vi "Google - Raw Stock Data - Parse.vi"(0 "Raw Stock Data":string, 3 "error in":errorcluster) -> (7 "Stock Data":T1, 10 "error out":errorcluster)   [LabVIEW 2011]
doc: "Parse the Raw Stock Data to a cluster structure.\n\nInputs:\n Raw Stock Data: Body of the HTTP request.\n Error in: Describes error conditions that occur before this node runs. This input provides standard error in functionality.\n\nOutputs:\n Stock Data: Parsed Stock Data\n Symbol\n Name\n Price\n Change\n Change %\n Volume: N/A\n Error out: Contains error information. This output provides standard error out functionality."
uses:
  Stock Data Control.ctl
panel:
  out "Raw Data":string
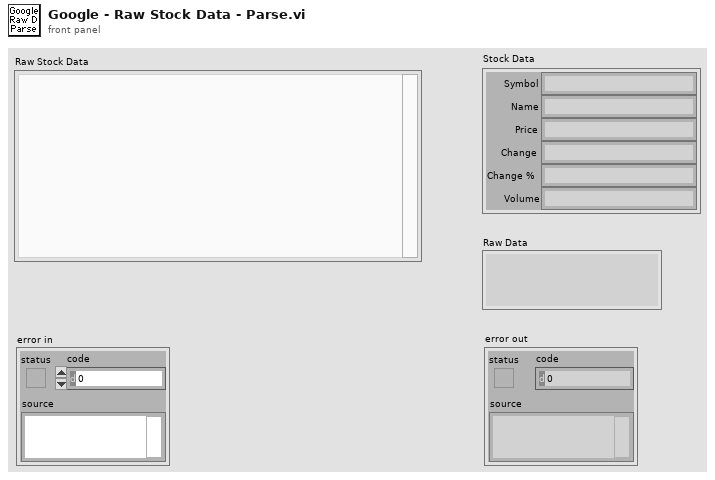
[diagram p1: front panel]
types:
  T1 = typedef "Stock Data Control.ctl" = cluster{"Symbol":string, "Name":string, "Price":string, "Change":string, "Change %":string, "Volume":string}
  T2 = cluster{"Symbol":string, "Name":string, "Price":string, "Change":string, "Change %":string, "Volume":string}
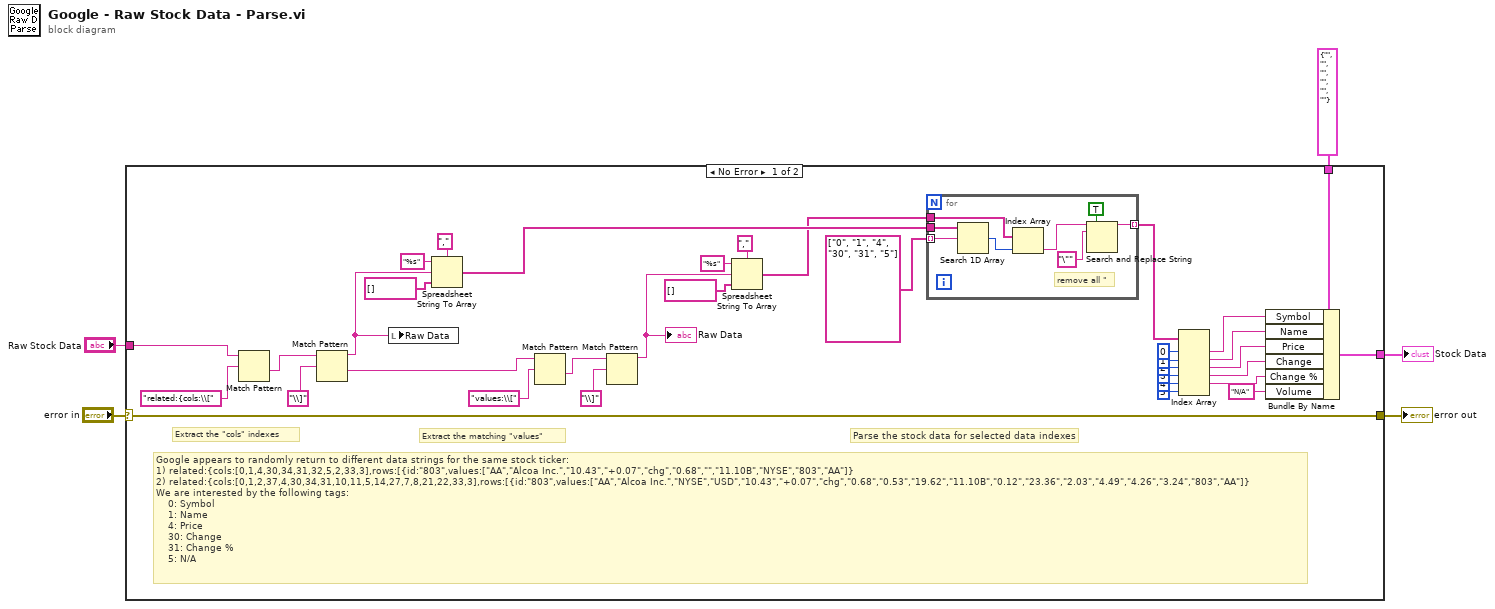
[diagram p0: block diagram]
diagram:
  n1 = case shown="No Error" "error in" {
    selector: "error in" -> [w40 w50]
    tunnel: [w40 w50] -> w4
    tunnel: "Raw Stock Data" -> [w22 _]
    tunnel: [w39 w49] -> w2
    tunnel: T2 {"Symbol"="", "Name"="", "Price"="", "Change"="", "Change %"="", "Volume"=""} ("Data") -> [w38 w49]
    frame No Error {
      # "Extract the matching \"values\""
      # "Extract the \"cols\" indexes"
      # "Parse the stock data for selected data indexes"
      # "Google appears to randomly return to different data strings for the same stock ticker:\n1) related:{cols:[0,1,4,30,34,31,32,5,2,33,3],rows:[{id:\"803\",values:[\"AA\",\"Alcoa Inc.\",\"10.43\",\"+0.07\",\"chg\",\"0.68\",\"\",\"11.10B\",\"NYSE\",\"803\",\"AA\"]}\n2) related:{cols:[0,1,2,37,4,30,34,31,10,11,5,14,27,7,8,21,22,33,3],rows:[{id:\"803\",values:[\"AA\",\"Alcoa Inc.\",\"NYSE\",\"USD\",\"10.43\",\"+0.07\",\"chg\",\"0.68\",\"0.53\",\"19.62\",\"11.10B\",\"0.12\",\"23.36\",\"2.03\",\"4.49\",\"4.26\",\"3.24\",\"803\",\"AA\"]}\nWe are interested by the following tags:\n    0: Symbol\n    1: Name\n    4: Price\n    30: Change\n    31: Change %\n    5: N/A"
      n2 = Match Pattern(string=w22, regular expression="related:{cols:\\[") -> (after substring=w23:string)  [unwired: 1 in, 3 out]
      n3 = Match Pattern(string=w23, regular expression="\\]") -> (before substring=w13:string, after substring=w21:string)  [unwired: 1 in, 2 out]
      n4 = local write "Raw Data"(w13) -> ()
      n5 = Spreadsheet String To Array(delimiter (Tab)=",", format string="%s", spreadsheet string=w13, array type (2D Dbl)=string[] []) -> (array=w12:string[])
      n6 = Match Pattern(string=w21, regular expression="values:\\[") -> (after substring=w29:string)  [unwired: 1 in, 3 out]
      n7 = Match Pattern(string=w29, regular expression="\\]") -> (before substring=w7:string)  [unwired: 1 in, 3 out]
      "Raw Data" <- w7
      n8 = Spreadsheet String To Array(delimiter (Tab)=",", format string="%s", spreadsheet string=w7, array type (2D Dbl)=string[] []) -> (array=w8:string[])
      n9 = for {
        tunnel: w12 -> [w48]
        tunnel: string[] ["0", "1", "4", "30", "31", "5"] -> [w47] mode=indexing
        tunnel: w8 -> [w45]
        tunnel: [w42] -> w17 mode=indexing
        # "remove all \""
        n10 = Search 1D Array(1D array=w48, element=w47) -> (index of element=w46:i32)  [unwired: 1 in]
        n11 = Index Array(array=w45, index=w46) -> (element=w44:string)
        n12 = Search and Replace String(replace all?=TRUE ("replace all? (F)"), input string=w44, search string="\"" ("format string")) -> (result string=w42:string)  [unwired: 5 in, 3 out]
      }
      n13 = Index Array(array=w17, index #1=0 ("index"), index #2=1 ("index"), index #3=2 ("index"), index #4=3 ("index"), index #5=4 ("index"), index #6=5 ("index")) -> (element #1=w33:string, element #2=w32:string, element #3=w31:string, element #4=w30:string, element #5=w25:string)  [unwired: 1 out]
      n14 = Bundle By Name(cluster=w38, "Symbol"=w33, "Name"=w32, "Price"=w31, "Change"=w30, "Change %"=w25, "Volume"="N/A") -> (w39:T2)
    }
    frame Error {
    }
  }
  "error out" <- w4
  "Stock Data" <- w2
